vi "Read Config.vi"(8 "error in":errorcluster, 11 "Data":T1={"Config"={"Hipot"={"COM PORT"=0, "AC to Pack"={"Mode"=0, "Voltage Level"=1000.0, "Low Limit"=0.0, "Hi Limit"=0.001, "ARC Limit"=0.0, "Step"=1.0, "Ramp Time "=0.0, "Test Time "=3.0}, "AC to Pack IR"={"Mode"=0, "Voltage Level IR"=1000.0, "Low Limit"=10000000.0, "Hi Limit"=0.001, "Real Current Limit"=0.0, "Step"=1.0, "Ramp Time "=0.0, "Test Time "=3.0}, "Pack to Case"={"Mode"=0, "Voltage Level"=1000.0, "Low Limit"=10000000.0, "Hi Limit"=0.0, "ARC Limit"=1.0, "Step"=0.0, "Ramp Time "=3.0, "Test Time "=3.0}, "Pack to Case IR"={"Mode"=0, "Voltage Level IR"=1000.0, "Low Limit"=10000000.0, "Hi Limit"=0.0, "Real Current Limit"=0.0, "Step"=1.0, "Ramp Time "=0.0, "Test Time "=3.0}}, "62150H-600 Supply"={"IVI Resource Name"=""}, "6320X E Load Heater"={"IVI Resource Name"=""}, "6320X E Load Compressor"={"IVI Resource Name"=""}, "6320X E Load DCDC"={"IVI Resource Name"=""}, "12061 DMM"={"IVI Resource Name"=""}, "17040 Pack Regen"={"IVI Resource Name"=""}}, "Test Data Ref"=refnum, "Current State Ref"=refnum, "Hipot Ref"=refnum, "Contactors Ref"=refnum, "Equipment Status Ref"=refnum, "TX Packet Info Ref"=refnum, "Pcap Cluster Ref"=refnum, "Eth Adapter ID Ref"=refnum, "Pass/Fail Results Ref"=refnum, "Sequence to Send Ref"=refnum, "Transmit Btn Ref"=refnum, "HW Handles Ref"=refnum, "MPB Status Ref"=refnum, "HVIL Source Ref"=refnum, "HVIL Readback Ref"=refnum, "Coolant Flow Ref"=refnum, "Coolant Temp Ref"=refnum, "Chiller Valve Open % Ref"=refnum} {"Config"."Hipot"."Pack to Case IR"."Test Time" min=0.0 max=999.0 step=0.1 format="%.1f"; "Config"."Hipot"."Pack to Case IR"."Ramp Time" min=0.0 max=999.0 step=0.1 format="%.1f"; "Config"."Hipot"."Pack to Case IR"."Step" min=1.0 max=99.0 step=1.0; "Config"."Hipot"."Pack to Case IR"."Real Current Limit" min=0.0 max=0.03 step=1e-06 format="%.2p"; "Config"."Hipot"."Pack to Case IR"."Voltage Level IR" min=100.0 max=1000.0 step=2.0; "Config"."Hipot"."Pack to Case IR"."Hi Limit" min=0.0 max=50000000000.0 step=10000.0 format="%.2p"; "Config"."Hipot"."Pack to Case IR"."Low Limit" min=100000.0 max=50000000000.0 step=10000.0 format="%.2p"; "Config"."Hipot"."Pack to Case IR"."Mode" items=["AC", "DC", "IR"]; "Config"."Hipot"."Pack to Case"."Test Time" min=0.0 max=999.0 step=0.1 format="%.1f"; "Config"."Hipot"."Pack to Case"."Ramp Time" min=0.0 max=999.0 step=0.1 format="%.1f"; "Config"."Hipot"."Pack to Case"."Step" min=1.0 max=99.0 step=1.0; "Config"."Hipot"."Pack to Case"."ARC Limit" min=0.0 max=0.015 step=1e-06 format="%.2p"; "Config"."Hipot"."Pack to Case"."Hi Limit" min=1e-06 max=0.03 step=1e-06 format="%.2p"; "Config"."Hipot"."Pack to Case"."Low Limit" min=0.0 max=0.03 step=1e-06 format="%.2p"; "Config"."Hipot"."Pack to Case"."Voltage Level" min=100.0 max=6000.0 step=2.0; "Config"."Hipot"."Pack to Case"."Mode" items=["AC", "DC", "IR"]; "Config"."Hipot"."AC to Pack IR"."Test Time" min=0.0 max=999.0 step=0.1 format="%.1f"; "Config"."Hipot"."AC to Pack IR"."Ramp Time" min=0.0 max=999.0 step=0.1 format="%.1f"; "Config"."Hipot"."AC to Pack IR"."Step" min=1.0 max=99.0 step=1.0; "Config"."Hipot"."AC to Pack IR"."Real Current Limit" min=0.0 max=0.03 step=1e-06 format="%.2p"; "Config"."Hipot"."AC to Pack IR"."Voltage Level IR" min=100.0 max=1000.0 step=2.0; "Config"."Hipot"."AC to Pack IR"."Hi Limit" min=0.0 max=50000000000.0 step=10000.0 format="%.2p"; "Config"."Hipot"."AC to Pack IR"."Low Limit" min=100000.0 max=50000000000.0 step=10000.0 format="%.2p"; "Config"."Hipot"."AC to Pack IR"."Mode" items=["AC", "DC", "IR"]; "Config"."Hipot"."AC to Pack"."Test Time" min=0.0 max=999.0 step=0.1 format="%.1f"; "Config"."Hipot"."AC to Pack"."Ramp Time" min=0.0 max=999.0 step=0.1 format="%.1f"; "Config"."Hipot"."AC to Pack"."Step" min=1.0 max=99.0 step=1.0; "Config"."Hipot"."AC to Pack"."ARC Limit" min=0.0 max=0.015 step=1e-06 format="%.2p"; "Config"."Hipot"."AC to Pack"."Hi Limit" min=1e-06 max=0.03 step=1e-06 format="%.2p"; "Config"."Hipot"."AC to Pack"."Low Limit" min=0.0 max=0.03 step=1e-06 format="%.2p"; "Config"."Hipot"."AC to Pack"."Voltage Level" min=100.0 max=6000.0 step=2.0; "Config"."Hipot"."AC to Pack"."Mode" items=["AC", "DC", "IR"]}) -> (0 "error out":errorcluster, 2 "Config Read OK":bool, 3 "Data Out":T1={"Config"={"Hipot"={"COM PORT"=0, "AC to Pack"={"Mode"=0, "Voltage Level"=1000.0, "Low Limit"=0.0, "Hi Limit"=0.001, "ARC Limit"=0.0, "Step"=1.0, "Ramp Time "=0.0, "Test Time "=3.0}, "AC to Pack IR"={"Mode"=0, "Voltage Level IR"=1000.0, "Low Limit"=10000000.0, "Hi Limit"=0.001, "Real Current Limit"=0.0, "Step"=1.0, "Ramp Time "=0.0, "Test Time "=3.0}, "Pack to Case"={"Mode"=0, "Voltage Level"=1000.0, "Low Limit"=10000000.0, "Hi Limit"=0.0, "ARC Limit"=1.0, "Step"=0.0, "Ramp Time "=3.0, "Test Time "=3.0}, "Pack to Case IR"={"Mode"=0, "Voltage Level IR"=1000.0, "Low Limit"=10000000.0, "Hi Limit"=0.0, "Real Current Limit"=0.0, "Step"=1.0, "Ramp Time "=0.0, "Test Time "=3.0}}, "62150H-600 Supply"={"IVI Resource Name"=""}, "6320X E Load Heater"={"IVI Resource Name"=""}, "6320X E Load Compressor"={"IVI Resource Name"=""}, "6320X E Load DCDC"={"IVI Resource Name"=""}, "12061 DMM"={"IVI Resource Name"=""}, "17040 Pack Regen"={"IVI Resource Name"=""}}, "Test Data Ref"=refnum, "Current State Ref"=refnum, "Hipot Ref"=refnum, "Contactors Ref"=refnum, "Equipment Status Ref"=refnum, "TX Packet Info Ref"=refnum, "Pcap Cluster Ref"=refnum, "Eth Adapter ID Ref"=refnum, "Pass/Fail Results Ref"=refnum, "Sequence to Send Ref"=refnum, "Transmit Btn Ref"=refnum, "HW Handles Ref"=refnum, "MPB Status Ref"=refnum, "HVIL Source Ref"=refnum, "HVIL Readback Ref"=refnum, "Coolant Flow Ref"=refnum, "Coolant Temp Ref"=refnum, "Chiller Valve Open % Ref"=refnum} {"Config"."Hipot"."Pack to Case IR"."Test Time" min=0.0 max=999.0 step=0.1 format="%.1f"; "Config"."Hipot"."Pack to Case IR"."Ramp Time" min=0.0 max=999.0 step=0.1 format="%.1f"; "Config"."Hipot"."Pack to Case IR"."Step" min=1.0 max=99.0 step=1.0; "Config"."Hipot"."Pack to Case IR"."Real Current Limit" min=0.0 max=0.03 step=1e-06 format="%.2p"; "Config"."Hipot"."Pack to Case IR"."Voltage Level IR" min=100.0 max=1000.0 step=2.0; "Config"."Hipot"."Pack to Case IR"."Hi Limit" min=0.0 max=50000000000.0 step=10000.0 format="%.2p"; "Config"."Hipot"."Pack to Case IR"."Low Limit" min=100000.0 max=50000000000.0 step=10000.0 format="%.2p"; "Config"."Hipot"."Pack to Case IR"."Mode" items=["AC", "DC", "IR"]; "Config"."Hipot"."Pack to Case"."Test Time" min=0.0 max=999.0 step=0.1 format="%.1f"; "Config"."Hipot"."Pack to Case"."Ramp Time" min=0.0 max=999.0 step=0.1 format="%.1f"; "Config"."Hipot"."Pack to Case"."Step" min=1.0 max=99.0 step=1.0; "Config"."Hipot"."Pack to Case"."ARC Limit" min=0.0 max=0.015 step=1e-06 format="%.2p"; "Config"."Hipot"."Pack to Case"."Hi Limit" min=1e-06 max=0.03 step=1e-06 format="%.2p"; "Config"."Hipot"."Pack to Case"."Low Limit" min=0.0 max=0.03 step=1e-06 format="%.2p"; "Config"."Hipot"."Pack to Case"."Voltage Level" min=100.0 max=6000.0 step=2.0; "Config"."Hipot"."Pack to Case"."Mode" items=["AC", "DC", "IR"]; "Config"."Hipot"."AC to Pack IR"."Test Time" min=0.0 max=999.0 step=0.1 format="%.1f"; "Config"."Hipot"."AC to Pack IR"."Ramp Time" min=0.0 max=999.0 step=0.1 format="%.1f"; "Config"."Hipot"."AC to Pack IR"."Step" min=1.0 max=99.0 step=1.0; "Config"."Hipot"."AC to Pack IR"."Real Current Limit" min=0.0 max=0.03 step=1e-06 format="%.2p"; "Config"."Hipot"."AC to Pack IR"."Voltage Level IR" min=100.0 max=1000.0 step=2.0; "Config"."Hipot"."AC to Pack IR"."Hi Limit" min=0.0 max=50000000000.0 step=10000.0 format="%.2p"; "Config"."Hipot"."AC to Pack IR"."Low Limit" min=100000.0 max=50000000000.0 step=10000.0 format="%.2p"; "Config"."Hipot"."AC to Pack IR"."Mode" items=["AC", "DC", "IR"]; "Config"."Hipot"."AC to Pack"."Test Time" min=0.0 max=999.0 step=0.1 format="%.1f"; "Config"."Hipot"."AC to Pack"."Ramp Time" min=0.0 max=999.0 step=0.1 format="%.1f"; "Config"."Hipot"."AC to Pack"."Step" min=1.0 max=99.0 step=1.0; "Config"."Hipot"."AC to Pack"."ARC Limit" min=0.0 max=0.015 step=1e-06 format="%.2p"; "Config"."Hipot"."AC to Pack"."Hi Limit" min=1e-06 max=0.03 step=1e-06 format="%.2p"; "Config"."Hipot"."AC to Pack"."Low Limit" min=0.0 max=0.03 step=1e-06 format="%.2p"; "Config"."Hipot"."AC to Pack"."Voltage Level" min=100.0 max=6000.0 step=2.0; "Config"."Hipot"."AC to Pack"."Mode" items=["AC", "DC", "IR"]})   [LabVIEW 2020]
uses:
  controls/Data.ctl
  controls/Config.ctl
  controls/Hipot_DC_Config.ctl
  controls/Hipot_IR_Config.ctl
  controls/Test Data Table.ctl
  controls/Hipot.ctl
  controls/Contactors.ctl
  controls/Equipment Status.ctl
  MPB Port Encode Decode/SubVIs/TX Packet Info.ctl
  MPB Port Encode Decode/Ethernet Palette/Controls/VLAN Tag.ctl
  MPB Port Encode Decode/Ethernet Palette/Controls/Pcap Cluster.ctl
  controls/PassFailResults.ctl
  controls/HW Handles.ctl
  controls/MPB Status.ctl
  <vilib>/Utility/config.llb/Read Key (U32).vi
  <vilib>/Utility/config.llb/Read Key (I32).vi
  <vilib>/Utility/config.llb/NI_LVConfig.lvlib
  <vilib>/Utility/config.llb/Write Key (I32).vi
  MPB Port Encode Decode/Ethernet Palette.lvlib
panel:
  # "Other"
  # "AC Port Info"
  # "Battery Port Info"
  # "Fault Info"
  # "1"
  # "2"
  # "3"
  # "4"
  # "5"
  # "6"
  # "7"
  # "DC Bus Info"
  # "HAPS Info"
  # "Temps"
  # "1"
  # "2"
  # "Other"
  # "AC Port Info"
  # "Battery Port Info"
  # "Fault Info"
  # "1"
  # "2"
  # "3"
  # "4"
  # "5"
  # "6"
  # "7"
  # "DC Bus Info"
  # "HAPS Info"
  # "Temps"
  # "1"
  # "2"
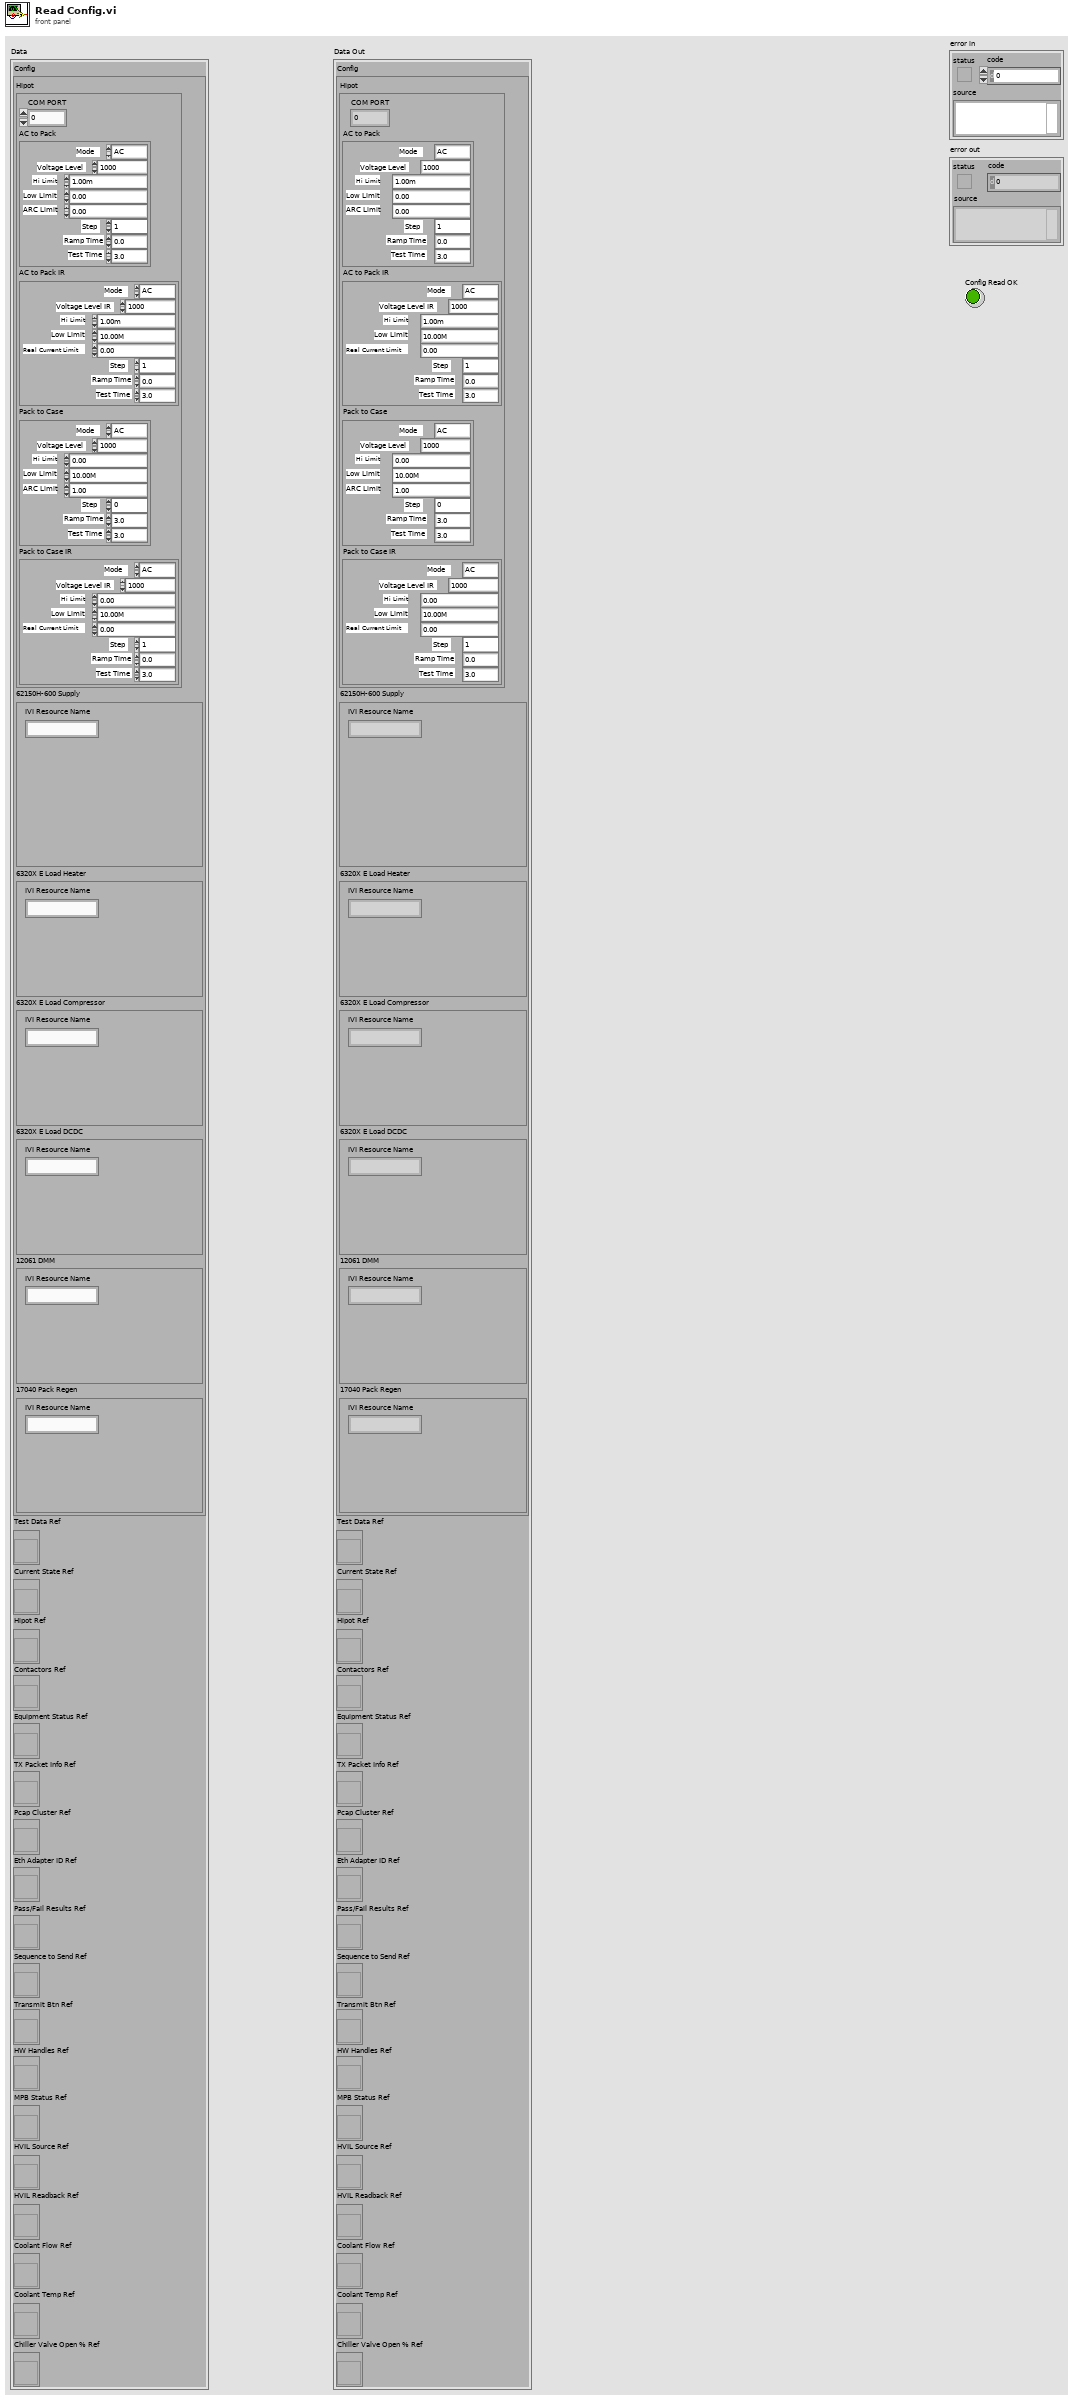
[diagram p1: front panel]
types:
  T1 = typedef "Data.ctl" = cluster{"Config":T2, "Test Data Ref":refnum<vi>, "Current State Ref":refnum<vi>, "Hipot Ref":refnum<vi>, "Contactors Ref":refnum<vi>, "Equipment Status Ref":refnum<vi>, "TX Packet Info Ref":refnum<vi>, "Pcap Cluster Ref":refnum<vi>, "Eth Adapter ID Ref":refnum<vi>, "Pass/Fail Results Ref":refnum<vi>, "Sequence to Send Ref":refnum<vi>, "Transmit Btn Ref":refnum<vi>, "HW Handles Ref":refnum<vi>, "MPB Status Ref":refnum<vi>, "HVIL Source Ref":refnum<vi>, "HVIL Readback Ref":refnum<vi>, "Coolant Flow Ref":refnum<vi>, "Coolant Temp Ref":refnum<vi>, "Chiller Valve Open % Ref":refnum<vi>}
  T2 = typedef "Config.ctl" = cluster{"Hipot":cluster{"COM PORT":u16, "AC to Pack":T3, "AC to Pack IR":T4, "Pack to Case":T3, "Pack to Case IR":T4}, "62150H-600 Supply":cluster{"IVI Resource Name":string}, "6320X E Load Heater":cluster{"IVI Resource Name":string}, "6320X E Load Compressor":cluster{"IVI Resource Name":string}, "6320X E Load DCDC":cluster{"IVI Resource Name":string}, "12061 DMM":cluster{"IVI Resource Name":string}, "17040 Pack Regen":cluster{"IVI Resource Name":string}}
  T3 = typedef "Hipot_DC_Config.ctl" = cluster{"Mode":u16, "Voltage Level":dbl, "Low Limit":dbl, "Hi Limit":dbl, "ARC Limit":dbl, "Step":dbl, "Ramp Time ":dbl, "Test Time ":dbl}
  T4 = typedef "Hipot_IR_Config.ctl" = cluster{"Mode":u16, "Voltage Level IR":dbl, "Low Limit":dbl, "Hi Limit":dbl, "Real Current Limit":dbl, "Step":dbl, "Ramp Time ":dbl, "Test Time ":dbl}
  T5 = typedef "NI_LVConfig.lvlib/Config Data RefNum.ctl" = refnum<k1>
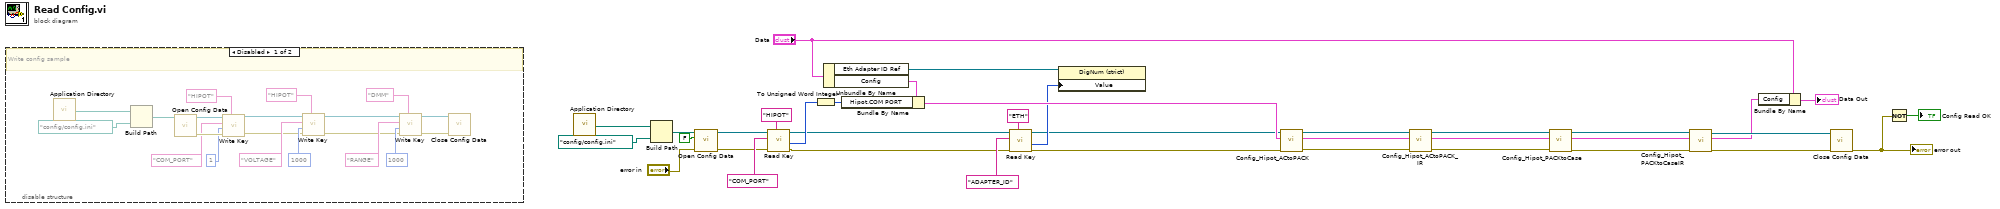
[diagram p0: block diagram]
diagram:
  n1 = disable-structure shown="Disabled" {
    frame Disabled {
      # "Write config sample"
      n2 = call <vilib>:"Application Directory.vi"() -> ("Application Directory"=w40:path)
      n3 = Build Path(base path=w40, name or relative path=path "config/config.ini") -> (appended path=w39:path)
      n4 = call <vilib>:"Open Config Data.vi"("configuration file path"=w39) -> ("error out"=w57:errorcluster, "refnum"=w38:T5)  [unwired: 8 in, 1 out]
      n5 = call-poly <vilib>:"Write Key.vi"("section"="HIPOT", "error in (no error)"=w57, "value"=1, "key"="COM_PORT", "refnum"=w38) -> ("error out"=w50:errorcluster, "refnum out"=w49:T5)  [unwired: 4 in, 1 out]
      n6 = call-poly <vilib>:"Write Key.vi"("section"="HIPOT", "error in (no error)"=w50, "value"=1000, "key"="VOLTAGE", "refnum"=w49) -> ("error out"=w45:errorcluster, "refnum out"=w44:T5)  [unwired: 4 in, 1 out]
      n7 = call-poly <vilib>:"Write Key.vi"("section"="DMM", "error in (no error)"=w45, "value"=1000, "key"="RANGE", "refnum"=w44) -> ("error out"=w43:errorcluster, "refnum out"=w42:T5)  [unwired: 4 in, 1 out]
      n8 = call <vilib>:"Close Config Data.vi"("error in (no error)"=w43, "refnum"=w42) -> ()  [unwired: 8 in, 2 out]
    }
    frame Enabled {
    }
  }
  n9 = call <vilib>:"Application Directory.vi"() -> ("Application Directory"=w36:path)
  n10 = Build Path(base path=w36, name or relative path=path "config/config.ini") -> (appended path=w37:path)
  n11 = call <vilib>:"Open Config Data.vi"("error in (no error)"="error in", "create file if necessary (T)"=FALSE, "configuration file path"=w37) -> ("error out"=w31:errorcluster, "refnum"=w34:T5)  [unwired: 6 in, 1 out]
  n12 = call-poly <vilib>:"Read Key.vi"("section"="HIPOT" ("key"), "error in (no error)"=w31, "key"="COM_PORT", "refnum"=w34) -> ("error out"=w4:errorcluster, "value"=w27:u32, "refnum out"=w5:T5)  [unwired: 4 in, 1 out]
  n13 = To Unsigned Word Integer(number=w27) -> (unsigned 16bit integer=w28:u16)
  n14 = Unbundle By Name("Data") -> ("Eth Adapter ID Ref"=w8:refnum<vi>, "Config"=w13:T2)
  n15 = Bundle By Name(cluster=w13, "Hipot.COM PORT"=w28) -> (w11:T2)
  n16 = call-poly <vilib>:"Read Key.vi"("section"="ETH" ("key"), "error in (no error)"=w4, "key"="ADAPTER_ID", "refnum"=w5) -> ("error out"=w2:errorcluster, "value"=w3:i32, "refnum out"=w1:T5)  [unwired: 4 in, 1 out]
  n17 = property class="DigNum (strict)"(reference=w8, "Value"=w3) -> ()  [unwired: 1 in, 2 out]
  n18 = call "Config_Hipot_ACtoPACK.vi"("error in (no error)"=w2, "Config in"=w11, "Config Ref In"=w1) -> ("error out"=w26:errorcluster, "Config Out"=w24:T2, "Config Ref Out"=w25:T5)  [unwired: 6 in]
  n19 = call "Config_Hipot_ACtoPACK_IR.vi"("error in (no error)"=w26, "Config in"=w24, "Config Ref In"=w25) -> ("error out"=w23:errorcluster, "Config Out"=w21:T2, "Config Ref Out"=w22:T5)  [unwired: 6 in]
  n20 = call "Config_Hipot_PACKtoCase.vi"("error in (no error)"=w23, "Config in"=w21, "Config Ref In"=w22) -> ("error out"=w20:errorcluster, "Config Out"=w18:T2, "Config Ref Out"=w19:T5)  [unwired: 6 in]
  n21 = call "Config_Hipot_PACKtoCaseIR.vi"("error in (no error)"=w20, "Config in"=w18, "Config Ref In"=w19) -> ("error out"=w17:errorcluster, "Config Out"=w12:T2, "Config Ref Out"=w16:T5)  [unwired: 6 in]
  n22 = Bundle By Name(cluster="Data", "Config"=w12) -> (→"Data Out":T1)
  n23 = call <vilib>:"Close Config Data.vi"("error in (no error)"=w17, "refnum"=w16) -> ("error out"=w15:errorcluster)  [unwired: 8 in, 1 out]
  "error out" <- w15
  n24 = Not(x=w15) -> (.not. x?=→"Config Read OK":bool)
